vi "BoatType.vi"() -> ()   [LabVIEW 2013]
panel:
  in  "Boat Type":T1(ring)
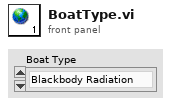
[diagram p1: front panel]
types:
  T1 = enum16{"Blackbody Radiation", "Little boats", "Simulation", "Damn Yankee"}
diagram:
